vi "Fetch Lists From Local DB.vi"(3 "error IN":errorcluster, 5 "Lookup Table Name":string) -> (0 "error OUT":errorcluster, 2 "recordset data":string[][](array[string]))   [LabVIEW 2010]
uses:
  <vilib>/addons/database/Connection.llb/DB Tools Open Connec (Path).vi
  <vilib>/addons/database/Connection.llb/Conn Execute.vi
  <vilib>/addons/database/Recordset.llb/Rec Destroy - Connection.vi
  <vilib>/addons/database/NI_Database_API.lvlib
panel:
  out "SP Call":string
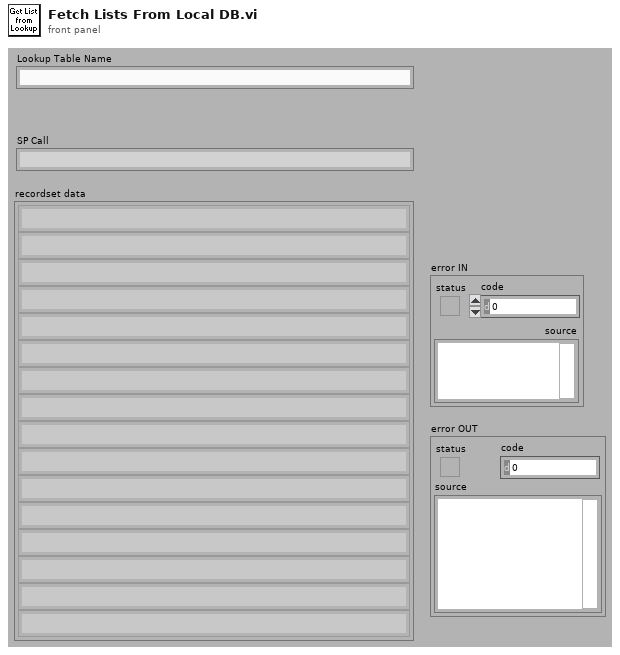
[diagram p1: front panel]
types:
  T1 = typedef "NI_Database_API.lvlib/Conn ObjectReference.ctl" = refnum<k1>
  T2 = typedef "NI_Database_API.lvlib/Rec ObjectReference.ctl" = refnum<k1>
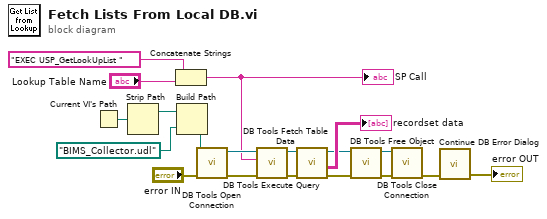
[diagram p0: block diagram]
diagram:
  n1 = Current VI's Path() -> (path=w7:path)
  n2 = Strip Path(path=w7) -> (stripped path=w6:path)  [unwired: 1 out]
  n3 = Concatenate Strings("EXEC USP_GetLookUpList " ("string"), "Lookup Table Name") -> (w2:string)
  "SP Call" <- w2
  n4 = Build Path(base path=w6, name or relative path=path "BIMS_Collector.udl" ("connectString")) -> (appended path=w4:path)
  n5 = call-poly <vilib>:"DB Tools Open Connection.vi"("error in (no error)"="error IN", "connection information"=w4) -> ("error out"=w12:errorcluster, "connection reference"=w10:T1)  [unwired: 3 in, 3 out]
  n6 = call-poly <vilib>:"DB Tools Execute Query.vi"("error in (no error)"=w12, "SQL query"=w2, "connection reference"=w10) -> ("error out"=w13:errorcluster, "recordset reference"=w9:T2)  [unwired: 1 in, 4 out]
  n7 = call <vilib>:"DB Tools Fetch Table Data.vi"("error in (no error)"=w13, "recordset reference"=w9) -> ("error out"=w14:errorcluster, "recordset data"=→"recordset data":string[][], "recordset reference out"=w8:T2)  [unwired: 3 out]
  n8 = call-poly <vilib>:"DB Tools Free Object.vi"("error in (no error)"=w14, "recordset reference"=w8) -> ("error out"=w15:errorcluster, "connection reference"=w11:T1)  [unwired: 8 out]
  n9 = call <vilib>:"DB Tools Close Connection.vi"("error in (no error)"=w15, "connection reference"=w11) -> ("error out"=w17:errorcluster)  [unwired: 5 out]
  n10 = call "Continue DB Error Dialog.vi"("error in (no error)"=w17) -> ("error out"=→"error OUT":errorcluster)  [unwired: 3 in, 2 out]
